vi "Signal InstConfig to Settings.vi"(8 "error in (no error)":errorcluster, 11 "Signal InstConfig":string) -> (0 "error out":errorcluster, 3 "Settings":cluster{"Channel":i32, "Current Limit Mode":T1})   [LabVIEW 2025, in "Interface Functions.lvlib"]
uses:
  Interface Functions/Interface Functions.lvlib
  Current Limit Mode--enum.ctl
  <vilib>/Utility/error.llb/Error Cluster From Error Code.vi
  <vilib>/ErrorRing/Error Ring.xnode
panel:
  # "Examples:\nChannel=2, CurrentLimitMode=Trip\nCurrentLimitMode=Regulate\nChannel=2\n\nDefaults:\nChannel=1,CurrentLimitMode=Regulate"
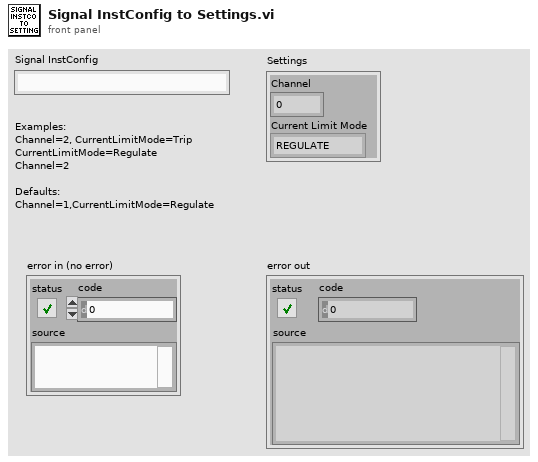
[diagram p1: front panel]
types:
  T1 = typedef "Interface Functions.lvlib/Current Limit Mode--enum.ctl" = enum16{"REGULATE", "TRIP"}
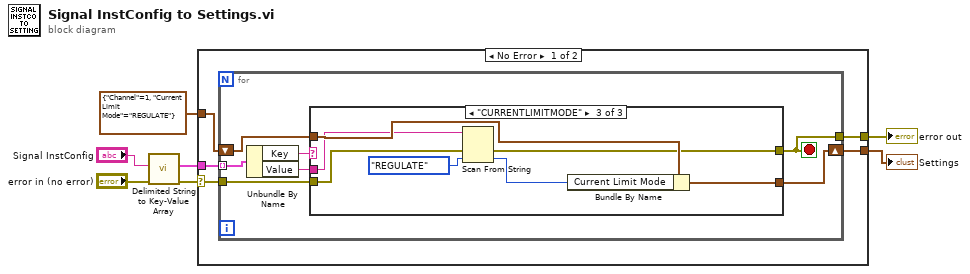
[diagram p0: block diagram]
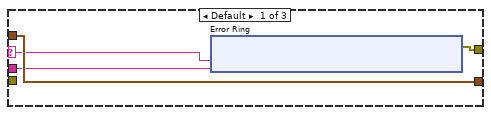
[diagram p2: hidden frame]
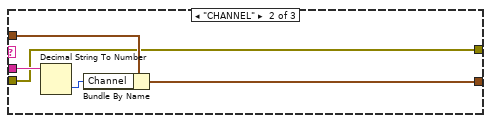
[diagram p3: hidden frame]
diagram:
  n1 = call "Delimited String to Key-Value Array.vi"("error in (no error)"="error in (no error)", "Delimited String"="Signal InstConfig") -> ("error out"=w3:errorcluster, "Key/Value Pairs"=w6:cluster{"Key":string, "Value":string}[])  [unwired: 8 in]
  n2 = case shown="No Error" w3 {
    selector: w3 -> [w8 w44]
    tunnel: w6 -> [w12 _]
    tunnel: cluster{"Channel":i32, "Current Limit Mode":T1} {"Channel"=1, "Current Limit Mode"=enum."REGULATE"} ("Settings") -> [w11 _]
    tunnel: [w10 _] -> w1
    tunnel: [w9 w44] -> w5
    frame No Error {
      n3 = for {
        tunnel: w12 -> [w19] mode=indexing
        shift-right: [w15] -> w10
        shift-left: w11 -> [w16]
        tunnel: [w13] -> w9
        tunnel: w8 -> [w14]
        stop <- w13 stop-if-true
        n4 = Unbundle By Name(w19) -> ("Key"=w18:string, "Value"=w17:string)
        n5 = case shown="\"CURRENTLIMITMODE\"" w18 {
          selector: w18 -> [w22 _ _]
          tunnel: w17 -> [w21 w34 w41]
          tunnel: w16 -> [w23 w36 w43]
          tunnel: [w23 w35 w42] -> w15
          tunnel: [w20 w32 w37] -> w13
          tunnel: w14 -> [_ w32 w38]
          frame Default {
            n6 = xnode "Error Ring"("parameter 0"=w22, "parameter 1"=w21) -> ("error out"=w20:errorcluster)
          }
          frame "CHANNEL" {
            n7 = Decimal String To Number(string=w34) -> (number=w33:i32)  [unwired: 2 in, 1 out]
            n8 = Bundle By Name(cluster=w36, "Channel"=w33) -> (w35:cluster{"Channel":i32, "Current Limit Mode":T1})
          }
          frame "CURRENTLIMITMODE" {
            n9 = Scan From String(input string=w41, error in=w38, default 1=Current_Limit_Mode--enum."REGULATE" ("Current Limit Mode")) -> (error out=w37:errorcluster, output 1=w39:T1)  [unwired: 2 in, 2 out]
            n10 = Bundle By Name(cluster=w43, "Current Limit Mode"=w39) -> (w42:cluster{"Channel":i32, "Current Limit Mode":T1})
          }
        }
      }
    }
    frame Error {
    }
  }
  "Settings" <- w1
  "error out" <- w5
